vi "Write Conf File.vi"(10 "Conf File":string, 11 "Update UI Status in":refnum<class "Update UI Status.lvclass">) -> (3 "Update UI Status out":refnum<class "Update UI Status.lvclass">)   [LabVIEW 2019, in "User Interface Process.lvlib" / "Update UI Status.lvclass"]
uses:
  Update UI Status.lvclass
  Update UI Status.lvclass/Update UI Status.ctl
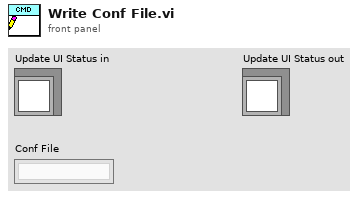
[diagram p1: front panel]
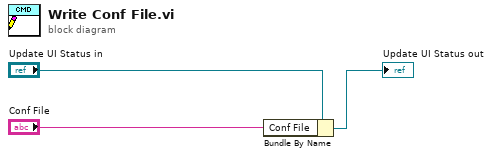
[diagram p0: block diagram]
diagram:
  n1 = Bundle By Name(cluster="Update UI Status in", "Conf File"="Conf File") -> (→"Update UI Status out":refnum<class "Update UI Status.lvclass">)
